vi "CmdCenter_RFSA_Meas.vi"(8 "error in (no error)":errorcluster, 11 "Message_Queues":T5) -> (0 "error out":errorcluster)   [LabVIEW 2014]
uses:
  15_DataManagement/Config_RFSA_Vertical.ctl
  15_DataManagement/Config_RFSA_IQ_Acq.ctl
  15_DataManagement/Config_RFSA_Spectrum_Acq.ctl
  15_DataManagement/Config_RFSG.ctl
  02_Controls/Message_Queues.ctl
  02_Controls/Message_Data_Ctl.ctl
  <vilib>/Utility/file.llb/Read From Spreadsheet File (string).vi
panel:
  in  "file path (dialog if empty)":path=path "C:/Gyuwon_Folder/SourceCodeFolder/1005_Gyu_RF_SourceProject_Msg/___SystemFiles/RecipeMode.ini"
  in  "Tab Control":enum32{"RFSG_Config", "RFSA_Config"}(tab)
  out "Config_RFSG":T1={"Carrier Frequency"=1500000000.0, "RF Power Level (dBm)"=-10.0, "SG External Gain (dBm)"=0.0, "Standard"=enum."LTE"} {"SG External Gain (dBm)" format="%#_6p"; "RF Power Level (dBm)" format="%#_6p"; "Carrier Frequency" format="%#_6p"}
  out "Config_RFSA_Vertical":T2={"Acquisition Type"=100, "Reference Level (dBm)"=-7.0, "External Gain (dB)"=0.0} {"External Gain (dB)" format="%#_13g"; "Reference Level (dBm)" format="%#_13g"; "Acquisition Type" items=["IQ"=100, "Spectrum"=101]}
  out "Config_RFSA_IQ_Acq":T3={"carrier frequency"=1500000000.0, "IQ rate (S/s)"=10000000.0, "samples per record"=1000000} {"IQ rate (S/s)" format="%#_6p"; "carrier frequency" format="%#_6p"}
  out "Config_RFSA_Spectrum_Acq":T4={"Resolution Bandwidth (Hz)"=10000.0, "Start Frequency (Hz)"=90000000.0, "Stop Frequency (Hz)"=110000000.0} {"Stop Frequency (Hz)" format="%#_6p"; "Start Frequency (Hz)" format="%#_6p"; "Resolution Bandwidth (Hz)" format="%#_6p"}
  out "Current_Message":string="Fetch_Complete"
  in  "Stop Button":bool
  in  "Start":bool
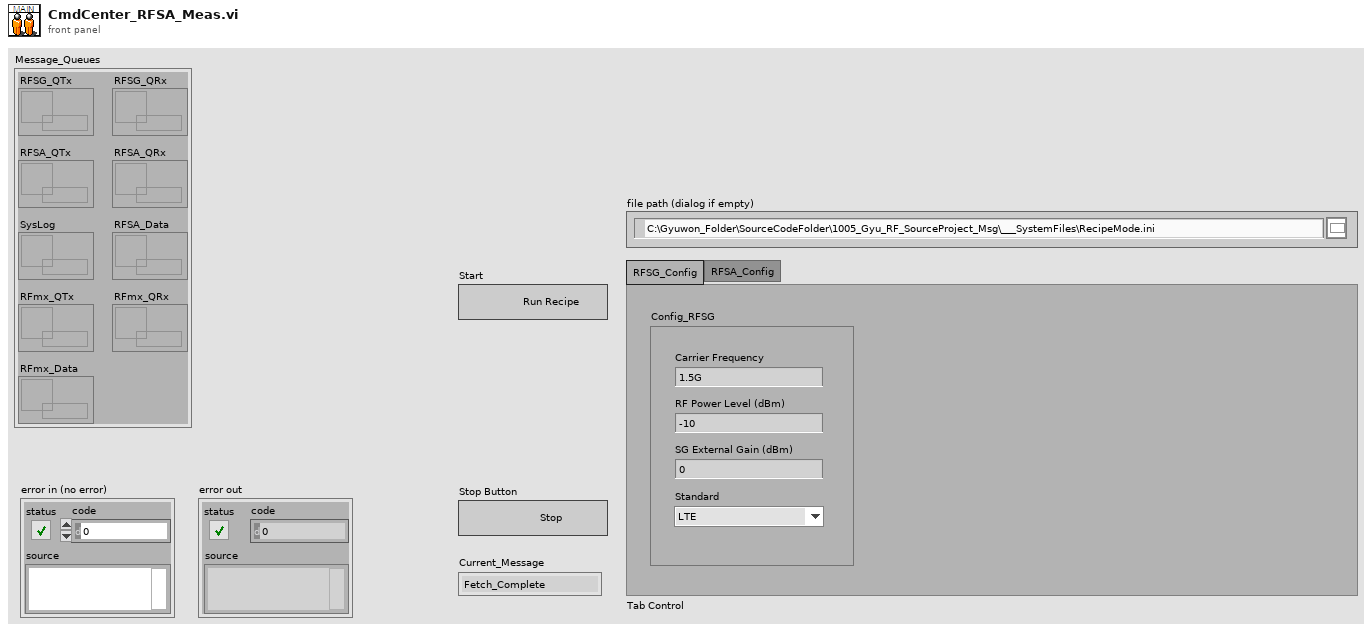
[diagram p1: front panel]
types:
  T1 = typedef "Config_RFSG.ctl" = cluster{"Carrier Frequency":dbl, "RF Power Level (dBm)":dbl, "SG External Gain (dBm)":dbl, "Standard":enum16{"LTE", "WCDMA", "GSM", "EDGE", "CW", "CWM"}}
  T2 = typedef "Config_RFSA_Vertical.ctl" = cluster{"Acquisition Type":i32, "Reference Level (dBm)":dbl, "External Gain (dB)":dbl}
  T3 = typedef "Config_RFSA_IQ_Acq.ctl" = cluster{"carrier frequency":dbl, "IQ rate (S/s)":dbl, "samples per record":i64}
  T4 = typedef "Config_RFSA_Spectrum_Acq.ctl" = cluster{"Resolution Bandwidth (Hz)":dbl, "Start Frequency (Hz)":dbl, "Stop Frequency (Hz)":dbl}
  T5 = typedef "Message_Queues.ctl" = cluster{"RFSG_QTx":refnum<queue>, "RFSG_QRx":refnum<queue>, "RFSA_QTx":refnum<queue>, "RFSA_QRx":refnum<queue>, "SysLog":refnum<queue>, "RFSA_Data":refnum<queue>, "RFmx_QTx":refnum<queue>, "RFmx_QRx":refnum<queue>, "RFmx_Data":refnum<queue>}
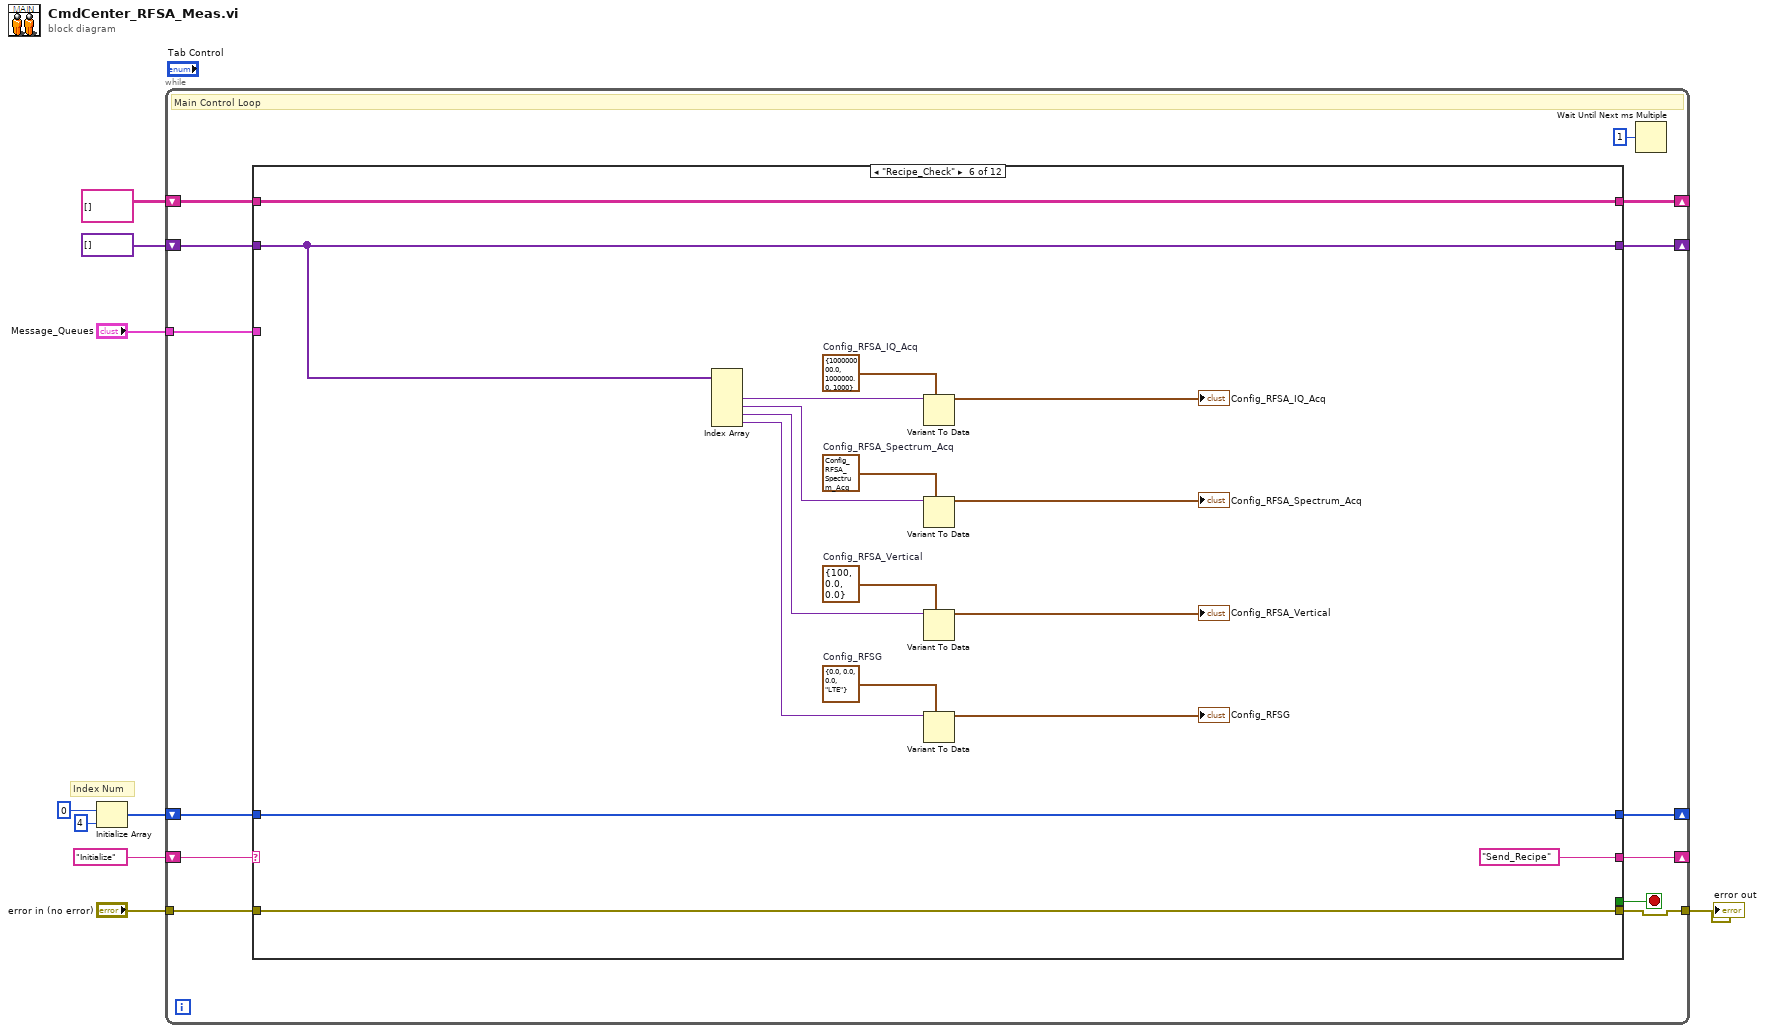
[diagram p0: block diagram]
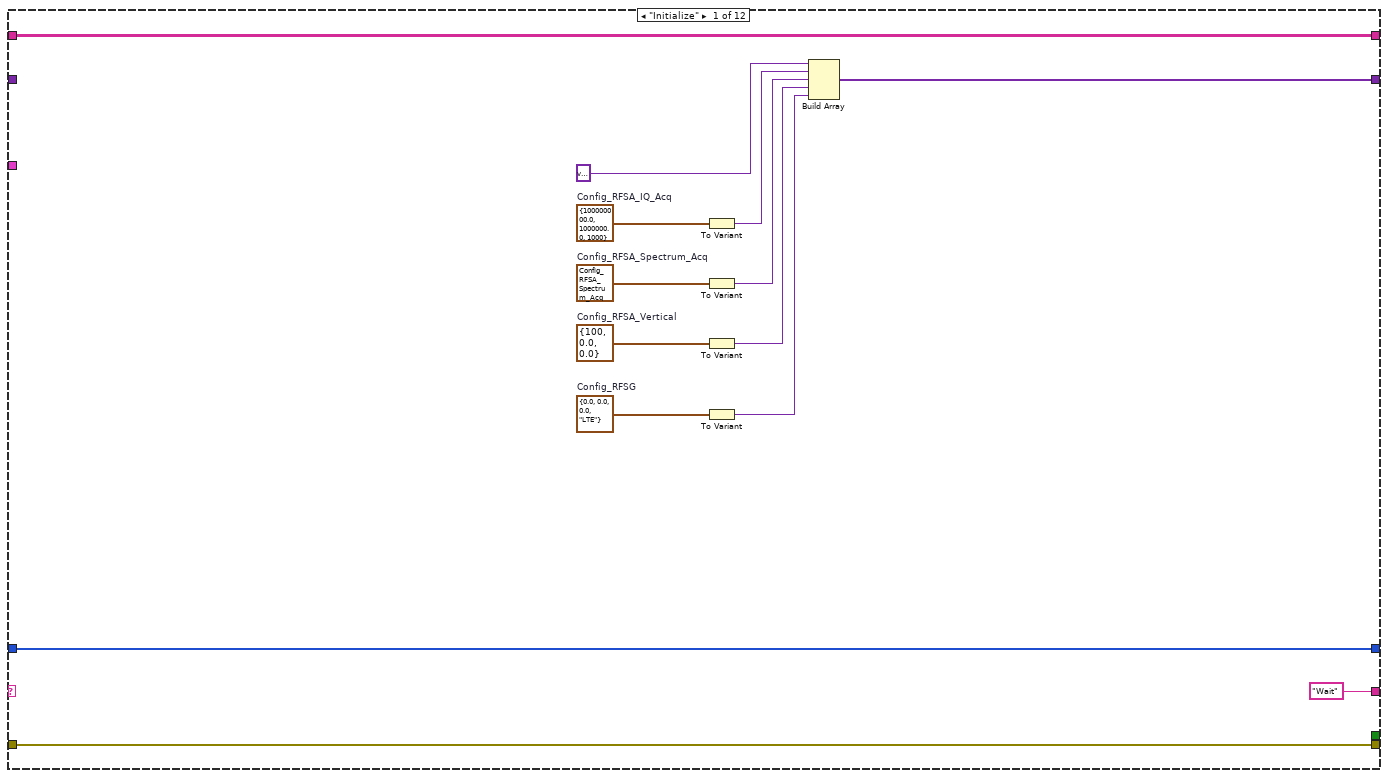
[diagram p2: hidden frame]
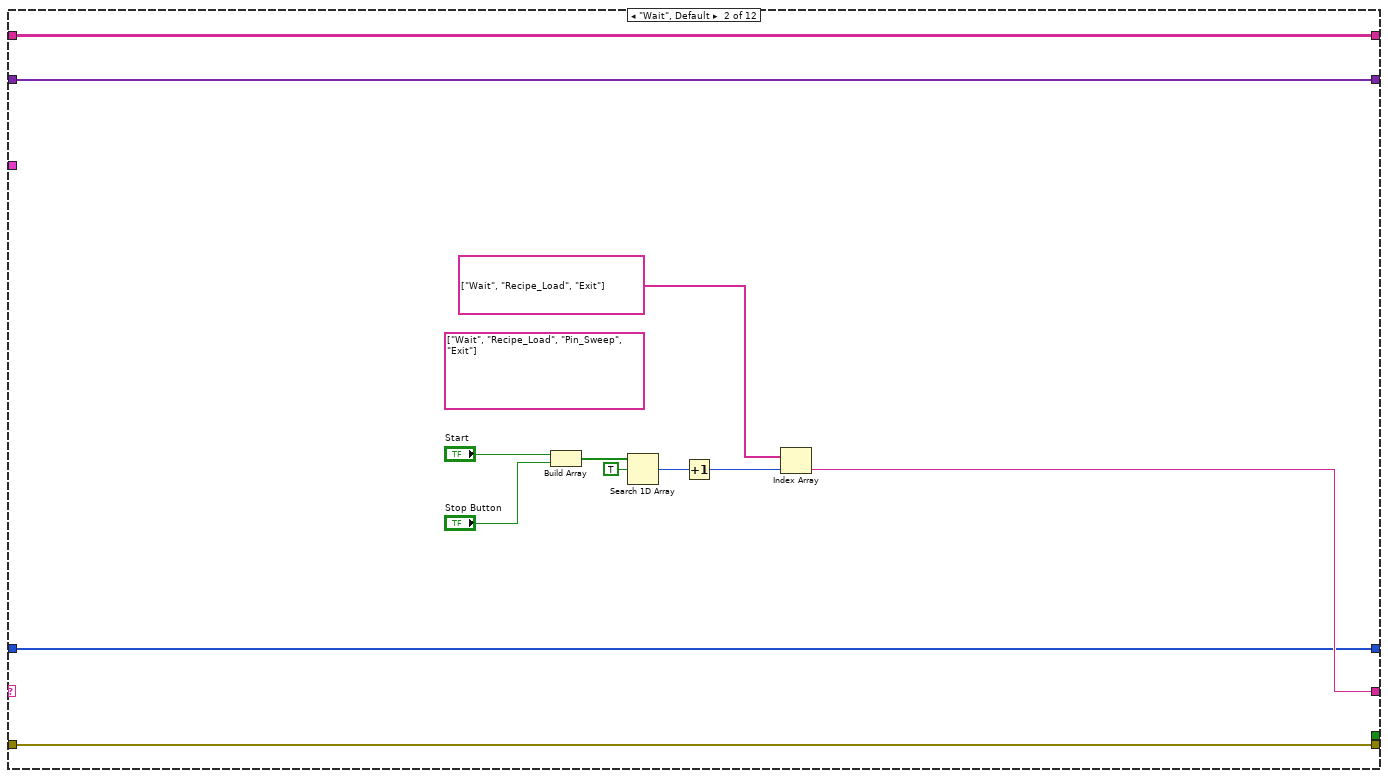
[diagram p3: hidden frame]
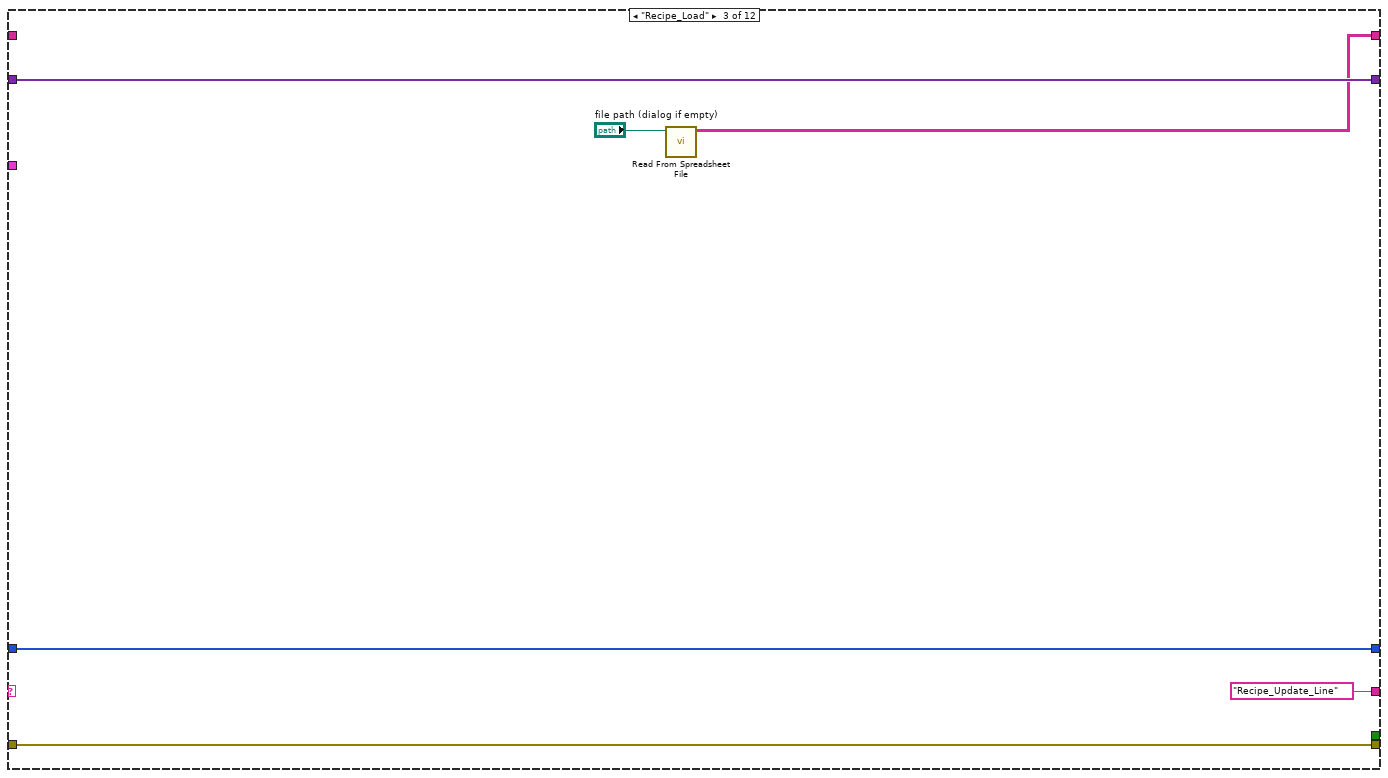
[diagram p4: hidden frame]
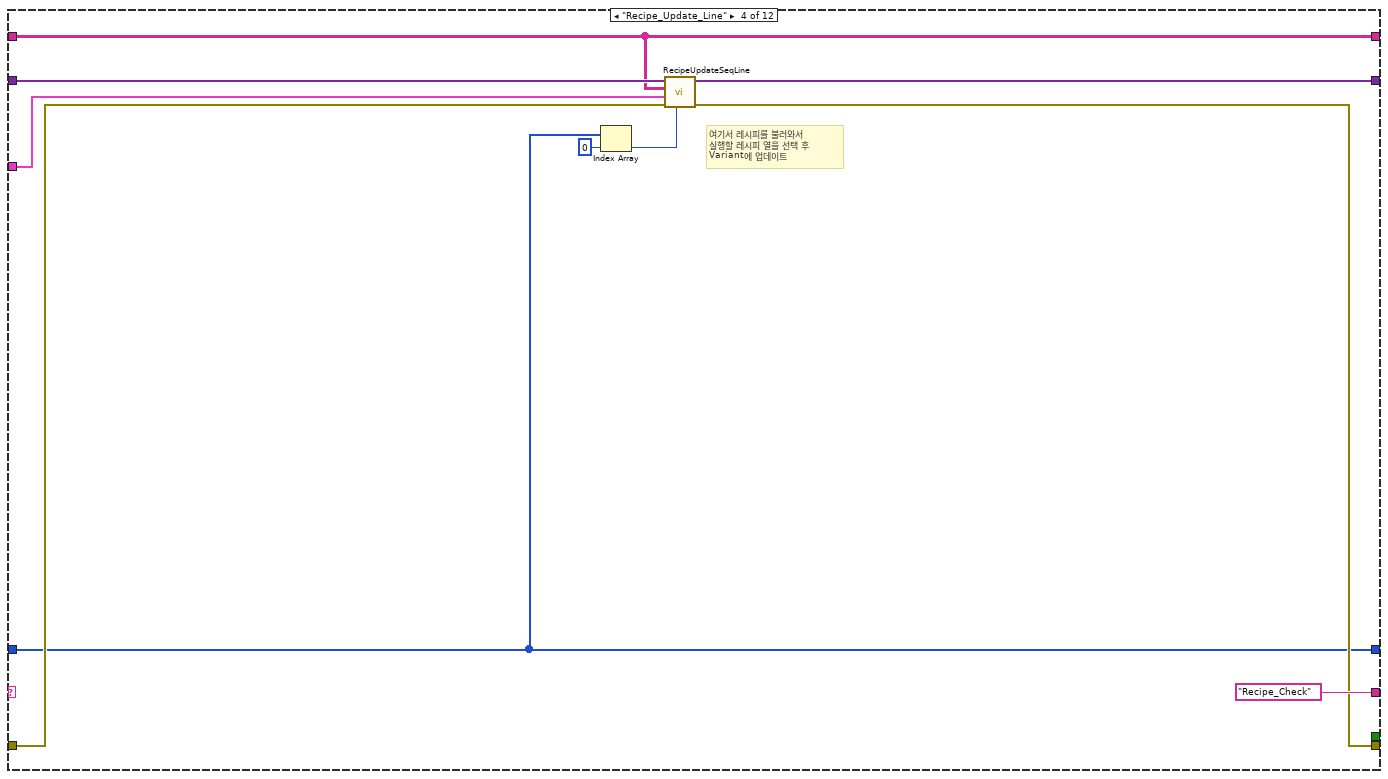
[diagram p5: hidden frame]
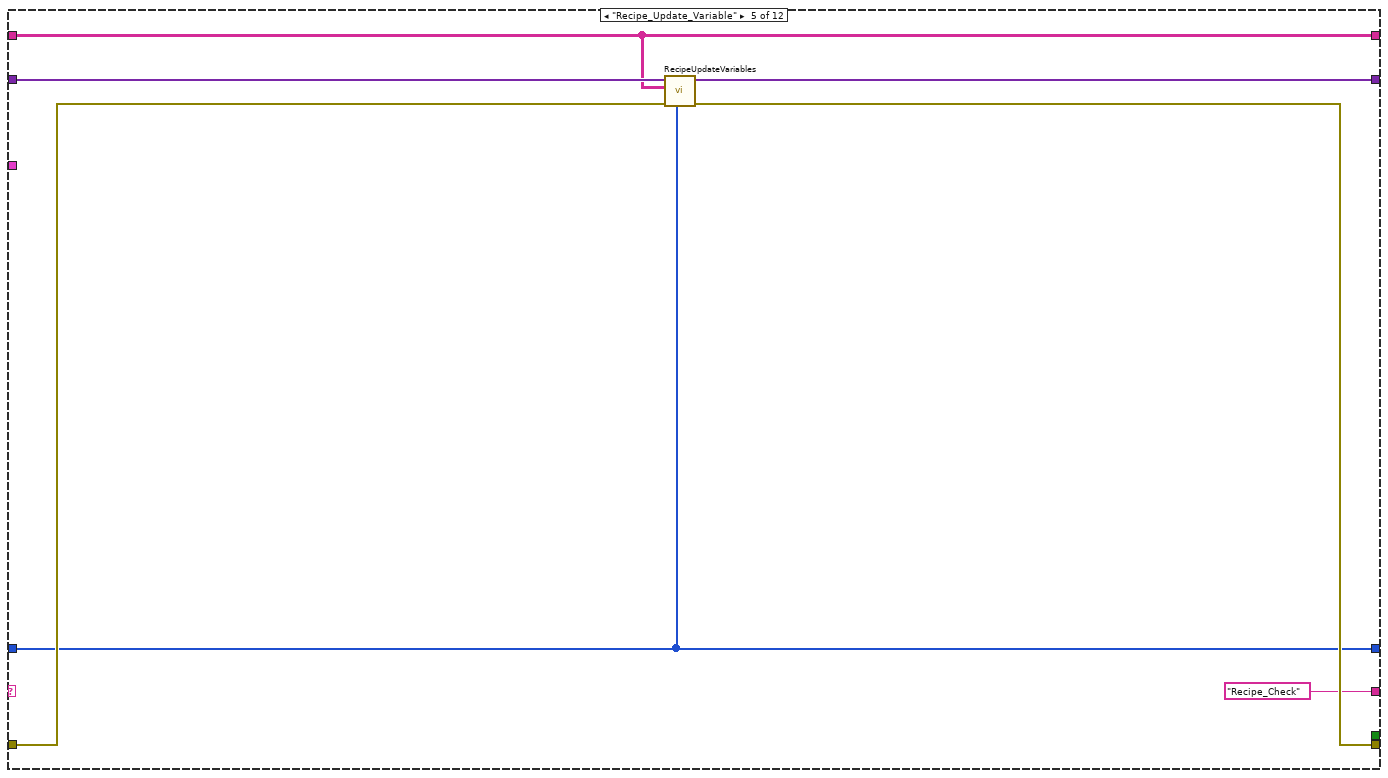
[diagram p6: hidden frame]
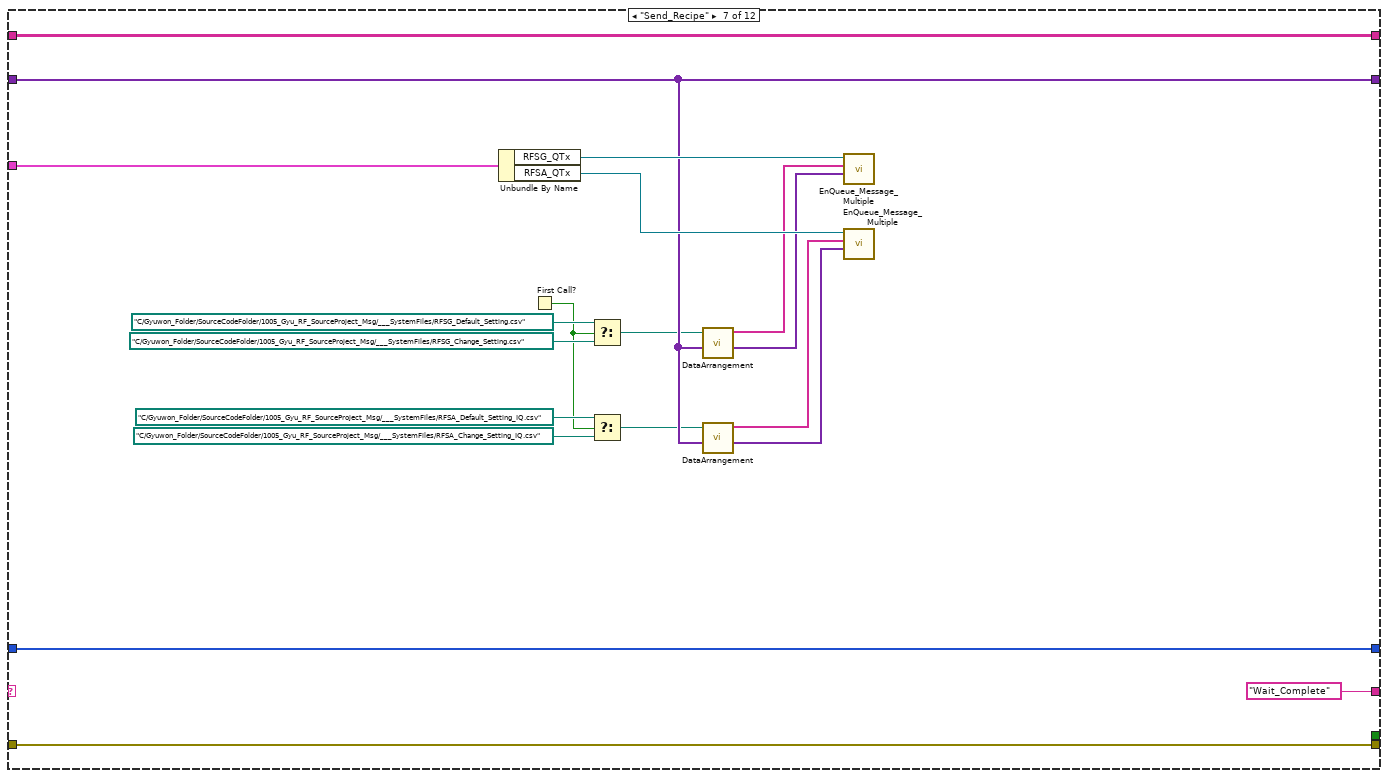
[diagram p7: hidden frame]
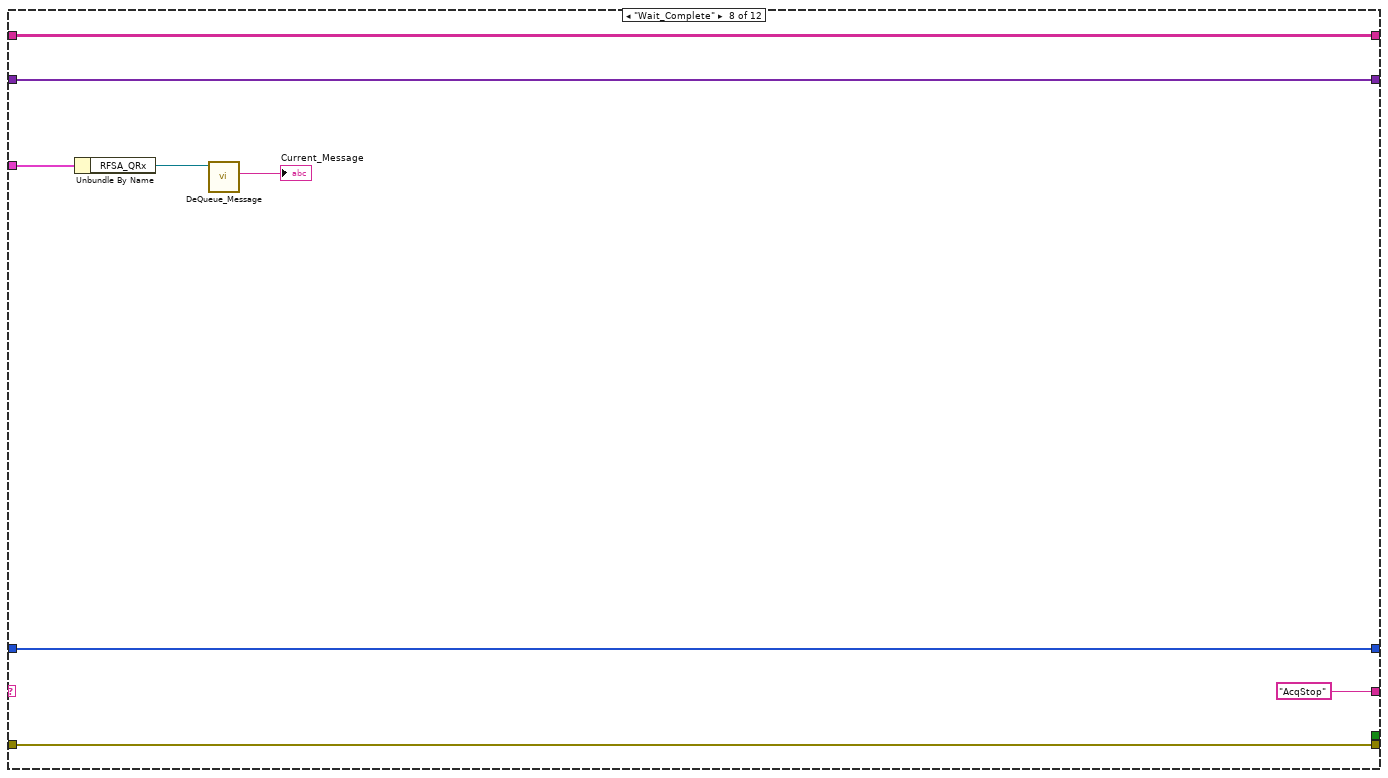
[diagram p8: hidden frame]
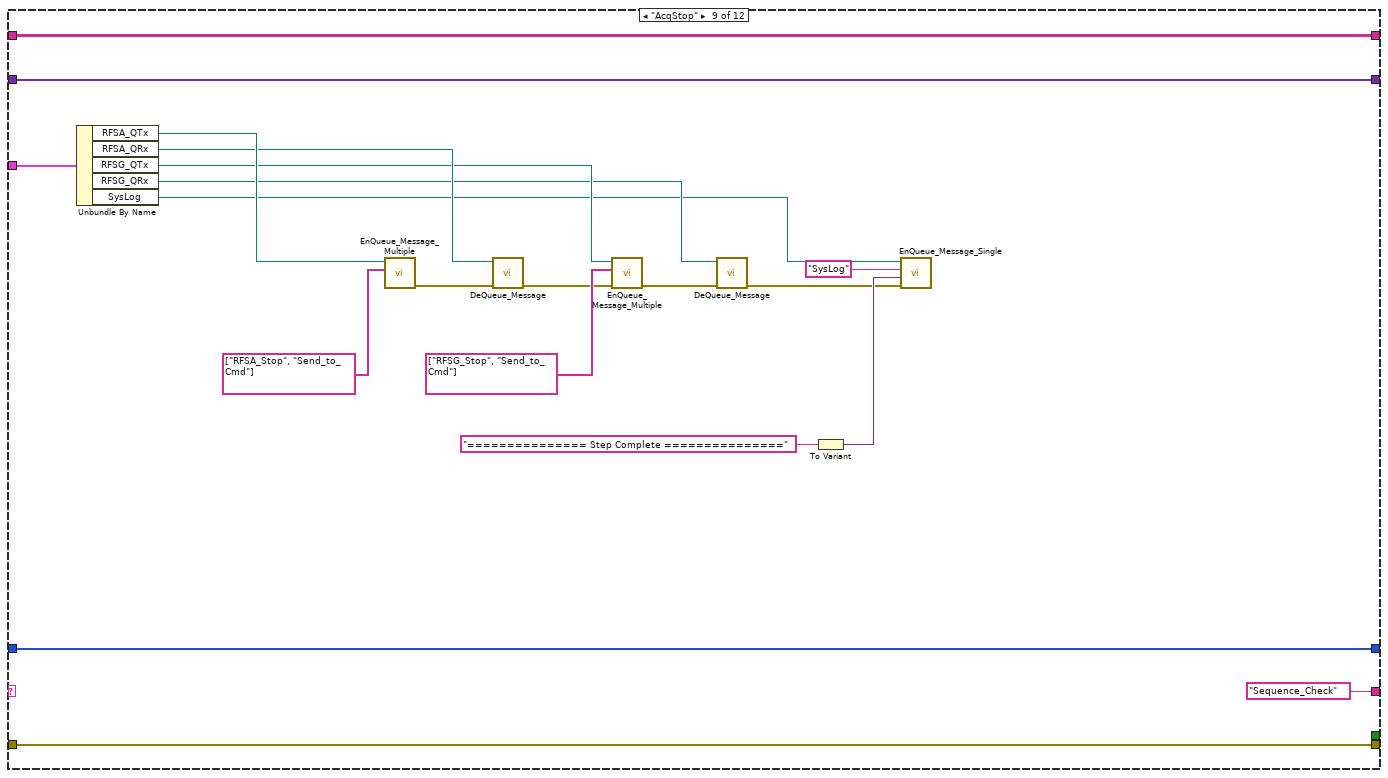
[diagram p9: hidden frame]
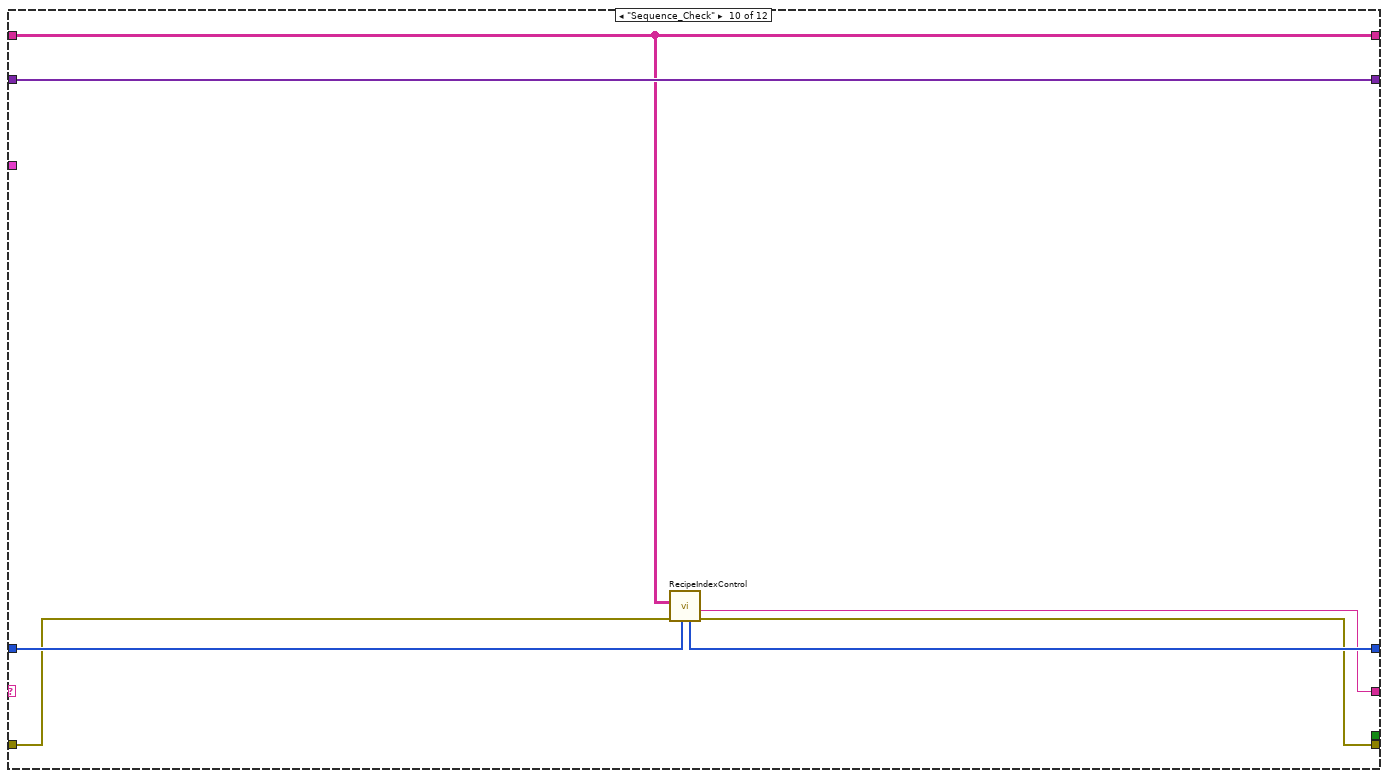
[diagram p10: hidden frame]
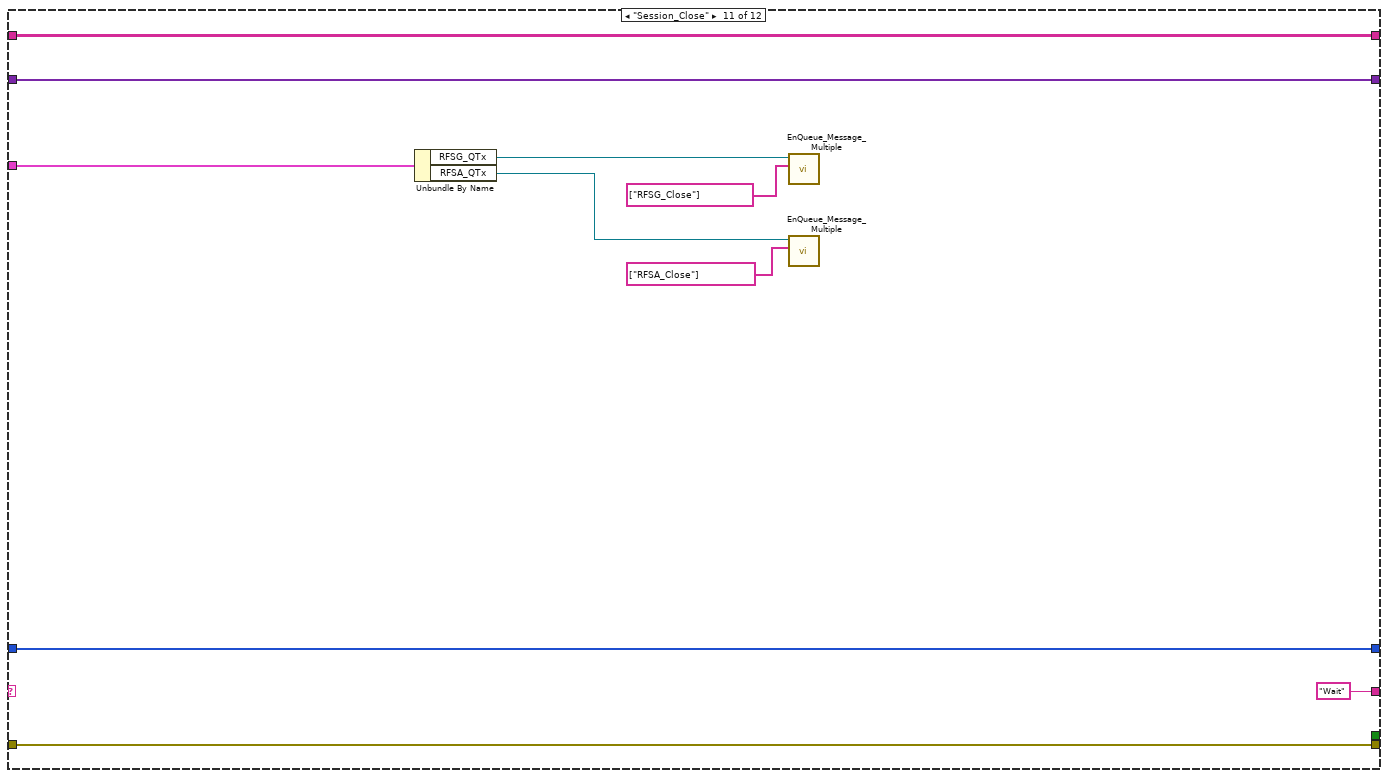
[diagram p11: hidden frame]
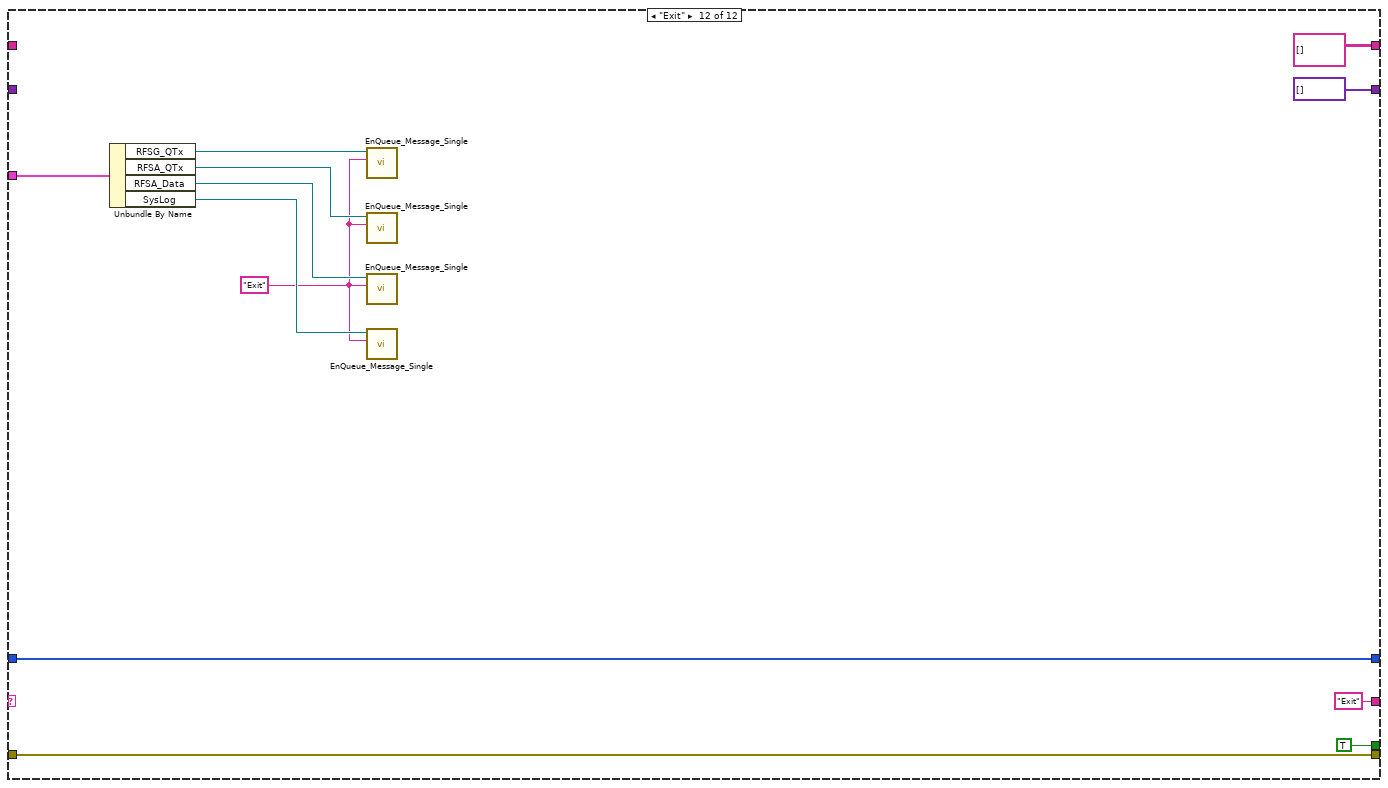
[diagram p12: hidden frame]
diagram:
  # "Index Num"
  n1 = Initialize Array(0, 4 ("dimension size")) -> (w1:i32[])
  n2 = while {
    tunnel: "error in (no error)" -> [w18]
    tunnel: [w21] -> w8
    tunnel: "Message_Queues" -> [w19]
    shift-right: [w16] -> _
    shift-left: "Initialize" -> [w20]
    shift-right: [w14] -> _
    shift-left: variant[] [] ("appended array") -> [w15]
    shift-right: [w13] -> _
    shift-left: string[][] [] ("all rows") -> [w12]
    shift-right: [w10] -> _
    shift-left: w1 -> [w11]
    stop <- w22 stop-if-true
    # "Main Control Loop"
    n3 = case shown="\"Recipe_Check\"" w20 {
      tunnel: w18 -> [w36 w48 w50 w61 w68 w87 w107 w115 w132 w139 w146 w163]
      tunnel: [_ _ _ _ _ _ _ _ _ _ _ TRUE] -> w22
      tunnel: [w36 w48 w50 w60 w67 w87 w107 w115 w132 w136 w146 w163] -> w21
      tunnel: w19 -> [_ _ _ w55 _ _ w106 w113 w134 _ w151 w161]
      tunnel: ["Wait" w42 "Recipe_Update_Line" "Recipe_Check" "Recipe_Check" "Send_Recipe" "Wait_Complete" "AcqStop" "Sequence_Check" w138 "Wait" "Exit"] -> w16
      tunnel: w15 -> [_ w41 w54 w63 w71 w86 w98 w110 w131 w142 w145 _]
      tunnel: [w25 w41 w54 w62 w70 w86 w98 w110 w131 w142 w145 variant[] [] ("appended array")] -> w14
      tunnel: [w24 w40 w52 w59 w69 w73 w97 w109 w130 w137 w144 string[][] [] ("all rows")] -> w13
      tunnel: w12 -> [w24 w40 _ w59 w69 w73 w97 w109 w130 w137 w144 _]
      tunnel: w11 -> [w23 w39 w49 w56 w65 w72 w96 w108 w129 w141 w143 w153]
      tunnel: [w23 w39 w49 w56 w65 w72 w96 w108 w129 w140 w143 w153] -> w10
      frame "Initialize" {
        w33 = T1 {"Carrier Frequency"=0.0, "RF Power Level (dBm)"=0.0, "SG External Gain (dBm)"=0.0, "Standard"=enum."LTE"}  # Config_RFSG
        w32 = T2 {"Acquisition Type"=100, "Reference Level (dBm)"=0.0, "External Gain (dB)"=0.0}  # Config_RFSA_Vertical
        w31 = T4 {"Resolution Bandwidth (Hz)"=10000.0, "Start Frequency (Hz)"=90000000.0, "Stop Frequency (Hz)"=110000000.0}  # Config_RFSA_Spectrum_Acq
        w34 = T3 {"carrier frequency"=100000000.0, "IQ rate (S/s)"=1000000.0, "samples per record"=1000}  # Config_RFSA_IQ_Acq
        n4 = To Variant(anything=w34) -> (Variant=w29:variant)
        n5 = To Variant(anything=w31) -> (Variant=w28:variant)
        n6 = To Variant(anything=w32) -> (Variant=w27:variant)
        n7 = To Variant(anything=w33) -> (Variant=w26:variant)
        n8 = Build Array(variant, w29, w28, w27, w26) -> (w25:variant[])
      }
      frame "Wait", Default {
        (unwired) string[] ["Wait", "Recipe_Load", "Pin_Sweep", "Exit"]
        n9 = Build Array("Start", "Stop Button") -> (w46:bool[])
        n10 = Search 1D Array(1D array=w46, element=TRUE) -> (index of element=w44:i32)  [unwired: 1 in]
        n11 = Increment(x=w44) -> (x+1=w43:i32)
        n12 = Index Array(array=string[] ["Wait", "Recipe_Load", "Exit"], index=w43) -> (element=w42:string)
      }
      frame "Recipe_Load" {
        n13 = call-poly <vilib>:"Read From Spreadsheet File.vi"("file path (dialog if empty)"="file path (dialog if empty)") -> ("all rows"=w52:string[][])  [unwired: 6 in, 4 out]
      }
      frame "Recipe_Update_Line" {
        # "여기서 레시피를 불러와서\n실행할 레시피 열을 선택 후\nVariant에 업데이트"
        n14 = Index Array(array=w56, index=0) -> (element=w57:i32)
        n15 = call "RecipeUpdateSeqLine.vi"("Seq_Index"=w57, "error in (no error)"=w61, "Message_Queues"=w55, "Recipe_Input"=w59, "DeviceSetup"=w63) -> ("error out"=w60:errorcluster, "DeviceSetup_Update"=w62:variant[])  [unwired: 5 in]
      }
      frame "Recipe_Update_Variable" {
        n16 = call "RecipeUpdateVariables.vi"("Index_List"=w65, "error in (no error)"=w68, "Recipe_Input"=w69, "DeviceSetup"=w71) -> ("error out"=w67:errorcluster, "DeviceSetup_Update"=w70:variant[])  [unwired: 6 in]
      }
      frame "Recipe_Check" {
        w83 = T1 {"Carrier Frequency"=0.0, "RF Power Level (dBm)"=0.0, "SG External Gain (dBm)"=0.0, "Standard"=enum."LTE"}  # Config_RFSG
        w81 = T2 {"Acquisition Type"=100, "Reference Level (dBm)"=0.0, "External Gain (dB)"=0.0}  # Config_RFSA_Vertical
        w82 = T4 {"Resolution Bandwidth (Hz)"=10000.0, "Start Frequency (Hz)"=90000000.0, "Stop Frequency (Hz)"=110000000.0}  # Config_RFSA_Spectrum_Acq
        w84 = T3 {"carrier frequency"=100000000.0, "IQ rate (S/s)"=1000000.0, "samples per record"=1000}  # Config_RFSA_IQ_Acq
        n17 = Index Array(array=w86) -> (element #2=w85:variant, element #3=w80:variant, element #4=w79:variant, element #5=w78:variant)  [unwired: 5 in, 1 out]
        n18 = Variant To Data(type=w84, Variant=w85) -> (data=→"Config_RFSA_IQ_Acq":T3)  [unwired: 1 in, 1 out]
        n19 = Variant To Data(type=w82, Variant=w80) -> (data=→"Config_RFSA_Spectrum_Acq":T4)  [unwired: 1 in, 1 out]
        n20 = Variant To Data(type=w81, Variant=w79) -> (data=→"Config_RFSA_Vertical":T2)  [unwired: 1 in, 1 out]
        n21 = Variant To Data(type=w83, Variant=w78) -> (data=→"Config_RFSG":T1)  [unwired: 1 in, 1 out]
      }
      frame "Send_Recipe" {
        n22 = Unbundle By Name(w106) -> ("RFSG_QTx"=w105:refnum<queue>, "RFSA_QTx"=w104:refnum<queue>)
        n23 = First Call?() -> (First Call?: T/F=w91:bool)
        n24 = Select(t=path "C:/Gyuwon_Folder/SourceCodeFolder/1005_Gyu_RF_SourceProject_Msg/___SystemFiles/RFSG_Default_Setting.csv" ("RFSG_List_1st"), s=w91, f=path "C:/Gyuwon_Folder/SourceCodeFolder/1005_Gyu_RF_SourceProject_Msg/___SystemFiles/RFSG_Change_Setting.csv" ("RFSG_List_1st")) -> (s? t:f=w90:path)
        n25 = Select(t=path "C:/Gyuwon_Folder/SourceCodeFolder/1005_Gyu_RF_SourceProject_Msg/___SystemFiles/RFSA_Default_Setting_IQ.csv" ("RFSA_List_1st"), s=w91, f=path "C:/Gyuwon_Folder/SourceCodeFolder/1005_Gyu_RF_SourceProject_Msg/___SystemFiles/RFSA_Change_Setting_IQ.csv" ("RFSA_List_1st")) -> (s? t:f=w89:path)
        n26 = call "DataArrangement.vi"("DataType"=w98, "file path (dialog if empty)"=w90) -> ("DataList"=w101:variant[], "CmdList"=w102:string[])  [unwired: 7 in, 1 out]
        n27 = call "DataArrangement.vi"("DataType"=w98, "file path (dialog if empty)"=w89) -> ("DataList"=w99:variant[], "CmdList"=w100:string[])  [unwired: 7 in, 1 out]
        n28 = call "EnQueue_Message_Multiple.vi"("Message Data Array"=w101, "Message Array"=w102, "Message_Queue"=w105) -> ()  [unwired: 7 in, 2 out]
        n29 = call "EnQueue_Message_Multiple.vi"("Message Data Array"=w99, "Message Array"=w100, "Message_Queue"=w104) -> ()  [unwired: 7 in, 2 out]
      }
      frame "Wait_Complete" {
        n30 = Unbundle By Name(w113) -> ("RFSA_QRx"=w112:refnum<queue>)
        n31 = call "DeQueue_Message.vi"("Message_Queue"=w112) -> ("Message"=→"Current_Message":string)  [unwired: 7 in, 3 out]
      }
      frame "AcqStop" {
        n32 = Unbundle By Name(w134) -> ("RFSA_QTx"=w128:refnum<queue>, "RFSA_QRx"=w127:refnum<queue>, "RFSG_QTx"=w125:refnum<queue>, "RFSG_QRx"=w123:refnum<queue>, "SysLog"=w122:refnum<queue>)
        n33 = call "EnQueue_Message_Multiple.vi"("Message Array"=string[] ["RFSA_Stop", "Send_to_Cmd"], "Message_Queue"=w128) -> ("error out"=w116:errorcluster)  [unwired: 8 in, 1 out]
        n34 = call "DeQueue_Message.vi"("error in (no error)"=w116, "Message_Queue"=w127) -> ("error out"=w117:errorcluster)  [unwired: 6 in, 3 out]
        n35 = call "EnQueue_Message_Multiple.vi"("error in (no error)"=w117, "Message Array"=string[] ["RFSG_Stop", "Send_to_Cmd"], "Message_Queue"=w125) -> ("error out"=w124:errorcluster)  [unwired: 7 in, 1 out]
        n36 = call "DeQueue_Message.vi"("error in (no error)"=w124, "Message_Queue"=w123) -> ("error out"=w118:errorcluster)  [unwired: 6 in, 3 out]
        n37 = To Variant(anything="=============== Step Complete ===============" ("Message")) -> (Variant=w119:variant)
        n38 = call "EnQueue_Message_Single.vi"("error in (no error)"=w118, "Message Data"=w119, "Message"="SysLog", "Message_Queue"=w122) -> ()  [unwired: 6 in, 2 out]
      }
      frame "Sequence_Check" {
        n39 = call "RecipeIndexControl.vi"("Index_List"=w141, "error in (no error)"=w139, "Recipe_Input"=w137) -> ("error out"=w136:errorcluster, "Status"=w138:string, "Index_List_out"=w140:i32[])  [unwired: 6 in]
      }
      frame "Session_Close" {
        n40 = Unbundle By Name(w151) -> ("RFSG_QTx"=w150:refnum<queue>, "RFSA_QTx"=w148:refnum<queue>)
        n41 = call "EnQueue_Message_Multiple.vi"("Message Array"=string[] ["RFSG_Close"], "Message_Queue"=w150) -> ()  [unwired: 8 in, 2 out]
        n42 = call "EnQueue_Message_Multiple.vi"("Message Array"=string[] ["RFSA_Close"], "Message_Queue"=w148) -> ()  [unwired: 8 in, 2 out]
      }
      frame "Exit" {
        w156 = "Exit" ("Message")
        n43 = Unbundle By Name(w161) -> ("RFSG_QTx"=w160:refnum<queue>, "RFSA_QTx"=w159:refnum<queue>, "RFSA_Data"=w158:refnum<queue>, "SysLog"=w157:refnum<queue>)
        n44 = call "EnQueue_Message_Single.vi"("Message"=w156, "Message_Queue"=w160) -> ()  [unwired: 8 in, 2 out]
        n45 = call "EnQueue_Message_Single.vi"("Message"=w156, "Message_Queue"=w159) -> ()  [unwired: 8 in, 2 out]
        n46 = call "EnQueue_Message_Single.vi"("Message"=w156, "Message_Queue"=w158) -> ()  [unwired: 8 in, 2 out]
        n47 = call "EnQueue_Message_Single.vi"("Message"=w156, "Message_Queue"=w157) -> ()  [unwired: 8 in, 2 out]
      }
    }
    n48 = Wait Until Next ms Multiple(millisecond multiple=u32 1) -> ()  [unwired: 1 out]
  }
  "error out" <- w8
